vi "Actors Test.vi"() -> ()   [LabVIEW 2020]
uses:
  Actors/Test/API/Test Actor API.lvclass
  Actors/Base Actor/API/Actor API.lvclass
  Actors/Logger/Actor/Logger Actor.lvclass
  Actors/Logger/API/Logger Actor API.lvclass
  RTAF Global References.vi
  C:/dev/PGS/2001 - TBCM/Source/RT/RTAF/Source/RTAF/Actors/Base Actor/API/Actor API.lvclass
  C:/dev/PGS/2001 - TBCM/Source/RT/RTAF/Source/RTAF/Actors/Logger/API/Logger Actor API.lvclass
  Actors/Logger/Actor/Config.ctl
  Actors/Test/Actor/Test Actor.lvclass
  C:/dev/PGS/2001 - TBCM/Source/RT/RTAF/Source/RTAF/Actors/Test/API/Test Actor API.lvclass
  Actors/Alarms Handler/Actor/Alarms Handler Actor.lvclass
  Actors/Alarms Handler/API/Alarms Handler Actor API.lvclass
  C:/dev/PGS/2001 - TBCM/Source/RT/RTAF/Source/RTAF/Actors/Alarms Handler/API/Alarms Handler Actor API.lvclass
  Actors/Alarms Handler/Actor/Config.ctl
  Actors/System Status/Actor/System Status Actor.lvclass
  Actors/System Status/API/System Status Actor API.lvclass
  C:/dev/PGS/2001 - TBCM/Source/RT/RTAF/Source/RTAF/Actors/System Status/API/System Status Actor API.lvclass
  Actors/Test/Actor/Count Behaviour.ctl
  <vilib>/Utility/RT CPU Load.ctl
  <vilib>/NI_Real-Time Target Support.lvlib
panel:
  out "CPU loads":T1[](array[typedef]) {"ISR (%)" format="%#.2f"; "Idle (%)" format="%#.2f"; "Background (%)" format="%#.2f"; "Normal (%)" format="%#.2f"; "Above Normal (%)" format="%#.2f"; "High (%)" format="%#.2f"; "Timed Structures (%)" format="%#.2f"; "Time Critical (%)" format="%#.2f"; "Total (%)" format="%#.2f"}
  out "Disk":T2
  out "Memory":T2
  in  "Add Alarm":bool
  in  "Error":errorcluster
  in  "Test Window State":T3(ring)
  in  "Alarm":string
  in  "Log Alarm":bool
  in  "Log Status":bool
  in  "Status":string
  in  "Alarms Handler Window State":T3(ring)
  in  "Logger Window State":T3(ring)
  out "Test Count":i32
  in  "Get Test Count":bool
  in  "Test Count Behaviour":T4
  # "Test"
  # "Logger"
  # "Alarms"
  # "System Status"
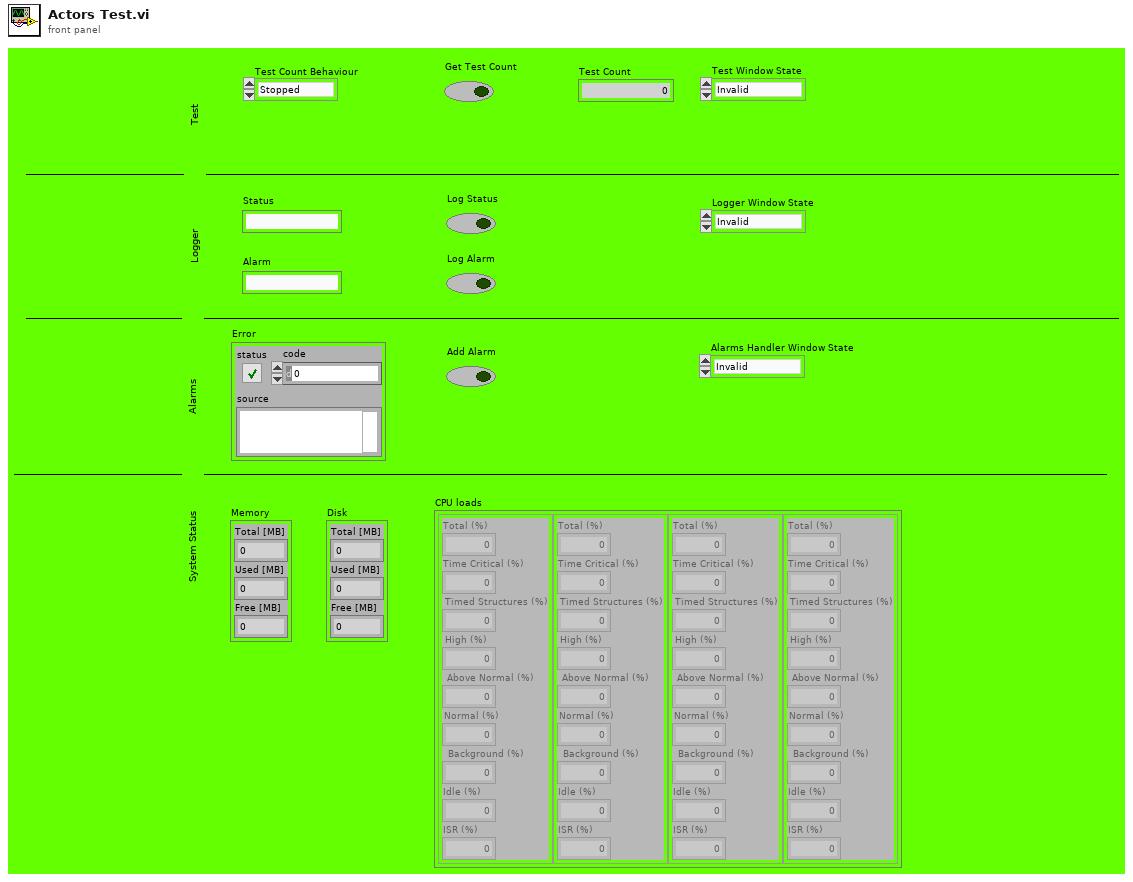
[diagram p1: front panel]
types:
  T1 = typedef "NI_Real-Time Target Support.lvlib/RT CPU Load.ctl" = cluster{"Total (%)":dbl, "Time Critical (%)":dbl, "Timed Structures (%)":dbl, "High (%)":dbl, "Above Normal (%)":dbl, "Normal (%)":dbl, "Background (%)":dbl, "Idle (%)":dbl, "ISR (%)":dbl}
  T2 = cluster{"Total [MB]":dbl, "Used [MB]":dbl, "Free [MB]":dbl}
  T3 = enum32{"Invalid", "Standard", "Closed", "Hidden", "Minimized", "Maximized"}
  T4 = typedef "Test Actor.lvclass/Count Behaviour.ctl" = enum16{"Stopped", "Up", "Down"}
  T5 = typedef "Alarms Handler Actor.lvclass/Config.ctl" = cluster{"Max Alarms Before Reset":i32}
  T6 = typedef "Logger Actor.lvclass/Config.ctl" = cluster{"Log Files Directory":path, "Max Lines Per File":i32}
  T7 = cluster{"System Status Actor":refnum<event-registration>}
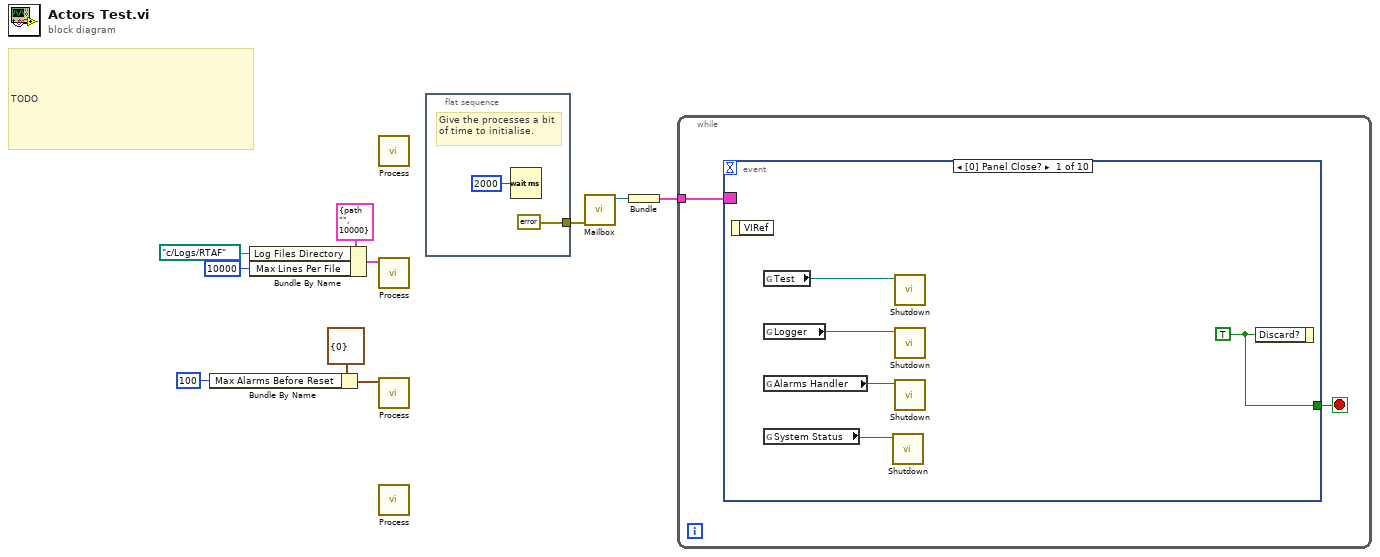
[diagram p0: block diagram]
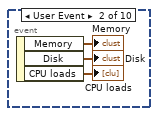
[diagram p2: hidden frame]
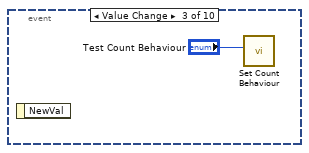
[diagram p3: hidden frame]
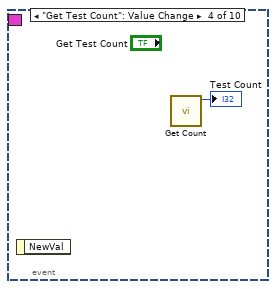
[diagram p4: hidden frame]
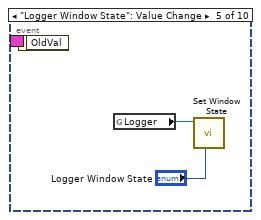
[diagram p5: hidden frame]
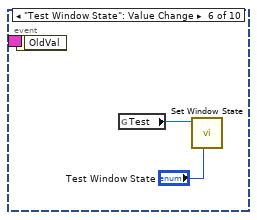
[diagram p6: hidden frame]
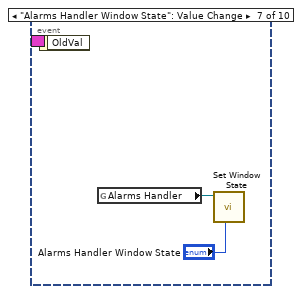
[diagram p7: hidden frame]
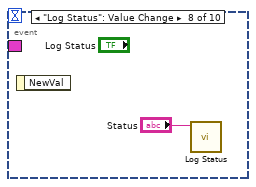
[diagram p8: hidden frame]
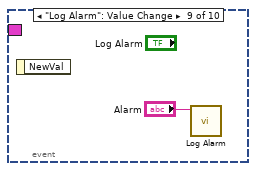
[diagram p9: hidden frame]
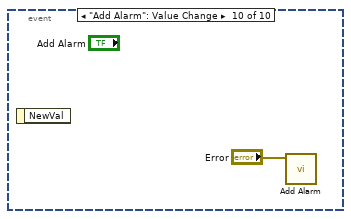
[diagram p10: hidden frame]
diagram:
  # "TODO"
  n1 = Bundle By Name(cluster=T5 {"Max Alarms Before Reset"=0} ("Config"), "Max Alarms Before Reset"=100) -> (w5:T5)
  n2 = Bundle By Name(cluster=T6 {"Log Files Directory"=path "", "Max Lines Per File"=10000} ("Initial Config"), "Log Files Directory"=path "c:/Logs/RTAF", "Max Lines Per File"=10000) -> (w9:T6)
  n3 = call "Process.vi"() -> ()  [unwired: 12 in]
  n4 = call "Process.vi"("Initial Config"=w9) -> ()  [unwired: 11 in]
  n5 = call "Process.vi"("Config"=w5) -> ()  [unwired: 11 in]
  n6 = call "Process.vi"() -> ()  [unwired: 12 in]
  n7 = flat-sequence {
    tunnel: [errorcluster {"status"=FALSE, "code"=0, "source"=""} ("error constant")] -> w1
    frame #0 {
      # "Give the processes a bit of time to initialise."
      n8 = Wait (ms)(milliseconds to wait=u32 2000) -> ()  [unwired: 1 out]
    }
  }
  n9 = call "Mailbox.vi"("error in (no error)"=w1) -> ("System Status Actor"=w3:refnum<event-registration>)  [unwired: 9 in, 1 out]
  n10 = Bundle("System Status Actor"=w3) -> (w2:T7)  [unwired: 1 in]
  n11 = while {
    tunnel: w2 -> [w13]
    stop <- w14 stop-if-true
    n12 = event shown="[0] Panel Close?" {
      selector: w13 -> [_ _ _ _ _ _ _ _ _ _]
      dyn-events: _ -> [_ _ _ _ _ _ _ _ _ _]
      timeout: _ -> [_ _ _ _ _ _ _ _ _ _]
      tunnel: [w19 _ _ _ _ _ _ _ _ _] -> w14
      event Panel Close? {
        w19 = TRUE ("Discard?")
        n13 = event-data() -> ()  [unwired: 1 in, 1 out]
        n14 = global read "RTAF Global References.vi" "Test"() -> (w17:refnum<class "Test Actor API.lvclass">)
        n15 = global read "RTAF Global References.vi" "Logger"() -> (w18:refnum<class "Logger Actor API.lvclass">)
        n16 = global read "RTAF Global References.vi" "Alarms Handler"() -> (w16:refnum<class "Alarms Handler Actor API.lvclass">)
        n17 = global read "RTAF Global References.vi" "System Status"() -> (w15:refnum<class "System Status Actor API.lvclass">)
        n18 = call "Shutdown.vi"("Actor API"=w15) -> ()  [unwired: 10 in, 1 out]
        n19 = call "Shutdown.vi"("Actor API"=w17) -> ()  [unwired: 10 in, 1 out]
        n20 = call "Shutdown.vi"("Actor API"=w18) -> ()  [unwired: 10 in, 1 out]
        n21 = call "Shutdown.vi"("Actor API"=w16) -> ()  [unwired: 10 in, 1 out]
        n22 = event-data("Discard?"=w19) -> ()  [unwired: 1 in, 1 out]
      }
      event User Event {
        n23 = event-data() -> ("Memory"=→"Memory":T2, "Disk"=→"Disk":T2, "CPU loads"=→"CPU loads":T1[])  [unwired: 1 in]
      }
      event Value Change {
        n24 = event-data() -> ()  [unwired: 1 in, 1 out]
        n25 = call "Set Count Behaviour.vi"("Count Behaviour"="Test Count Behaviour") -> ()  [unwired: 10 in, 1 out]
      }
      event "Get Test Count": Value Change {
        n26 = event-data() -> ()  [unwired: 1 in, 1 out]
        n27 = call "Get Count.vi"() -> ("Count"=→"Test Count":i32)  [unwired: 10 in, 1 out]
      }
      event "Logger Window State": Value Change {
        n28 = event-data() -> ()  [unwired: 1 in, 1 out]
        n29 = global read "RTAF Global References.vi" "Logger"() -> (w25:refnum<class "Logger Actor API.lvclass">)
        n30 = call "Set Window State.vi"("State"="Logger Window State", "Actor API"=w25) -> ()  [unwired: 9 in, 1 out]
      }
      event "Test Window State": Value Change {
        n31 = event-data() -> ()  [unwired: 1 in, 1 out]
        n32 = global read "RTAF Global References.vi" "Test"() -> (w28:refnum<class "Test Actor API.lvclass">)
        n33 = call "Set Window State.vi"("State"="Test Window State", "Actor API"=w28) -> ()  [unwired: 9 in, 1 out]
      }
      event "Alarms Handler Window State": Value Change {
        n34 = event-data() -> ()  [unwired: 1 in, 1 out]
        n35 = global read "RTAF Global References.vi" "Alarms Handler"() -> (w29:refnum<class "Alarms Handler Actor API.lvclass">)
        n36 = call "Set Window State.vi"("State"="Alarms Handler Window State", "Actor API"=w29) -> ()  [unwired: 9 in, 1 out]
      }
      event "Log Status": Value Change {
        n37 = event-data() -> ()  [unwired: 1 in, 1 out]
        n38 = call "Log Status.vi"("Message"="Status") -> ()  [unwired: 10 in, 1 out]
      }
      event "Log Alarm": Value Change {
        n39 = event-data() -> ()  [unwired: 1 in, 1 out]
        n40 = call "Log Alarm.vi"("Message"="Alarm") -> ()  [unwired: 10 in, 1 out]
      }
      event "Add Alarm": Value Change {
        n41 = event-data() -> ()  [unwired: 1 in, 1 out]
        n42 = call "Add Alarm.vi"("Alarm"="Error") -> ()  [unwired: 10 in, 1 out]
      }
    }
  }
